vi "Determine State of Boat.vi"() -> (5 "State of Boat":T1(ring))   [LabVIEW 2012]
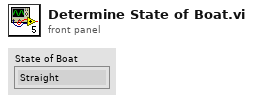
[diagram p1: front panel]
types:
  T1 = enum16{"Straight", "Turning", "Tacking", "Approach Maneuver", "Cross Wind (Tack)", "Cross Wind (Gybe)", "Turtle Mode", ""}
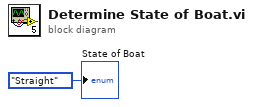
[diagram p0: block diagram]
diagram:
  "State of Boat" <- T1."Straight"
